vi "time_ceiling.vi"(2 "base (s)":dbl caption="基数 (s)", 3 "timestamp input":timestamp caption="时间标识输入") -> (0 "time diff (s)":dbl caption="时间差 (s)", 1 "timestamp output":timestamp caption="时间标识输出")   [LabVIEW 2015]
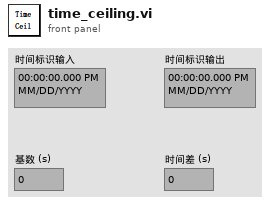
[diagram p1: front panel]
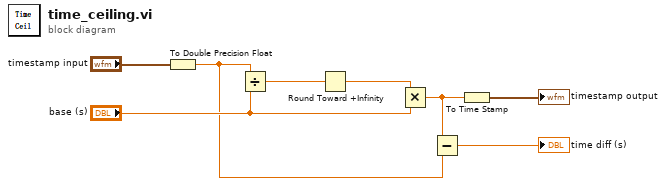
[diagram p0: block diagram]
diagram:
  n1 = To Double Precision Float(number="timestamp input") -> (double precision float=w1:dbl)
  n2 = Divide(x=w1, y="base (s)") -> (x/y=w7:dbl)
  n3 = Round Toward +Infinity(x=w7) -> (ceil(x): smallest int >= x=w6:dbl)
  n4 = Multiply(x=w6, y="base (s)") -> (x*y=w2:dbl)
  n5 = Subtract(x=w2, y=w1) -> (x-y=→"time diff (s)":dbl)
  n6 = To Time Stamp(1:w2) -> (0:→"timestamp output":timestamp)
